vi "XML Script - Tunnel.vi"(2 "out":i32=-1, 3 "default":bool, 4 "location":T1, 6 "name":string, 8 "offset":i32=1, 9 "prefix (name)":string, 10 "in":i32=-1) -> (5 "name (wire source)":string, 7 "XML Script Command - Tunnel":string)   [LabVIEW 2017]
uses:
  <vilib>/_script/XML Scripting/Structure Location.ctl
  <vilib>/_script/XML Scripting/XML Script Tag.ctl
  <vilib>/_script/XML Scripting/XML Script Attribute.ctl
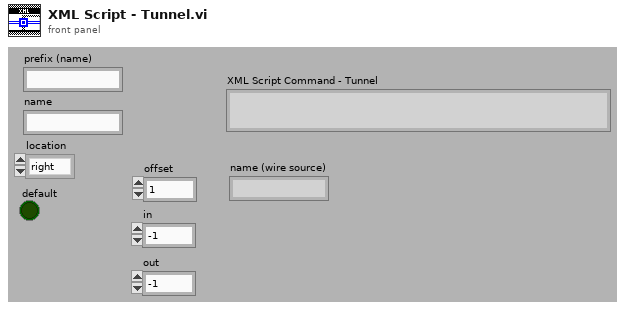
[diagram p1: front panel]
types:
  T1 = typedef "Structure Location.ctl" = enum16{"right", "left", "top", "bottom"}
  T2 = typedef "XML Script Attribute.ctl" = enum16{"name", "style", "path", "position", "in", "out", "width", "height", "index", "value", "default", "location", "offset", "typeindex", "size", "source", "destination", "indicator", "type", "controlname", "label", "conpaneidx", "mode", "description", "hasCondTerm", "linkIdentity", "caseselectortype", "concatInputs", "inName", "instantiationpath", "loopCondition", "IndexMode", "formulaInputs", "formulaOutputs", "msnFuncName", "msnIsDynamic", "msnIsODEUserFunction", "ignoreSearchDialog"}
  T3 = typedef "XML Script Tag.ctl" = enum16{"Script", "Function", "SubVI", "GrowableFunction", "Structure", "MultiframeStructure", "Frame", "Tunnel", "ShiftRegister", "Constant", "Control", "Terminal", "Wire", "StaticVIReference", "ControlTerminal", "CompoundArithmetic", "FlatSequence", "FlatSequenceFrame", "MathScriptCallByRef", "BuildArray", "GenericSubVI", "MathScriptNode"}
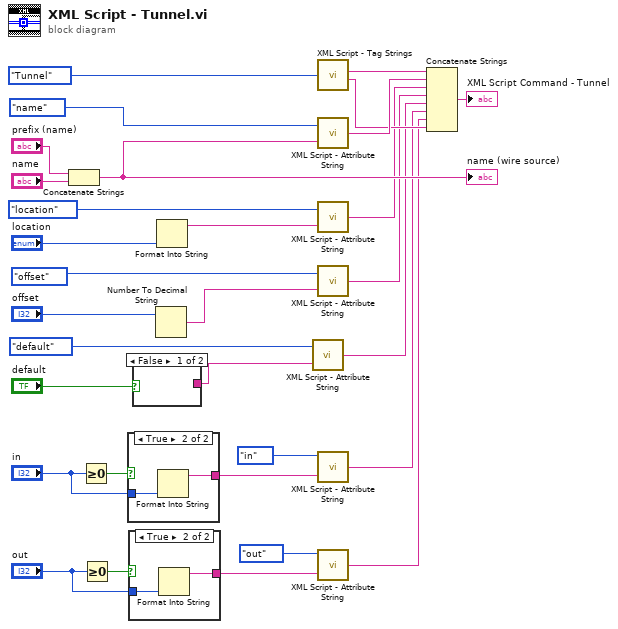
[diagram p0: block diagram]
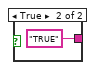
[diagram p2: hidden frame]
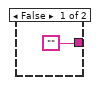
[diagram p3: hidden frame]
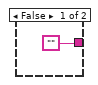
[diagram p4: hidden frame]
diagram:
  n1 = Concatenate Strings("prefix (name)", "name") -> (w21:string)
  "name (wire source)" <- w21
  n2 = Greater Or Equal To 0?(x="in") -> (x >= 0?=w11:bool)
  n3 = Greater Or Equal To 0?(x="out") -> (x >= 0?=w15:bool)
  n4 = case shown="True" w11 {
    tunnel: "in" -> [_ w34]
    tunnel: ["" w33] -> w13
    frame False {
    }
    frame True {
      n5 = Format Into String(w34) -> (resulting string=w33:string)  [unwired: 3 in, 1 out]
    }
  }
  n6 = case shown="True" w15 {
    tunnel: "out" -> [_ w37]
    tunnel: ["" w36] -> w17
    frame False {
    }
    frame True {
      n7 = Format Into String(w37) -> (resulting string=w36:string)  [unwired: 3 in, 1 out]
    }
  }
  n8 = case shown="False" "default" {
    tunnel: [_ "TRUE"] -> w2
    frame False {
    }
    frame True {
    }
  }
  n9 = Number To Decimal String(number="offset") -> (decimal integer string=w18:string)  [unwired: 1 in]
  n10 = Format Into String("location") -> (resulting string=w24:string)  [unwired: 3 in, 1 out]
  n11 = call <vilib>:"XML Script - Attribute String.vi"("Attribute String"=w2, "XML Script Attribute"=XML_Script_Attribute."default") -> ("XML Script - Attribute String"=w1:string)
  n12 = call <vilib>:"XML Script - Tag Strings.vi"("XML Script Tag"=XML_Script_Tag."Tunnel") -> ("XML String - Begin Tag"=w28:string, "XML String - End Tag"=w9:string)  [unwired: 2 in]
  n13 = call <vilib>:"XML Script - Attribute String.vi"("Attribute String"=w21, "XML Script Attribute"=XML_Script_Attribute."name") -> ("XML Script - Attribute String"=w26:string)
  n14 = call <vilib>:"XML Script - Attribute String.vi"("Attribute String"=w24, "XML Script Attribute"=XML_Script_Attribute."location") -> ("XML Script - Attribute String"=w5:string)
  n15 = call <vilib>:"XML Script - Attribute String.vi"("Attribute String"=w18, "XML Script Attribute"=XML_Script_Attribute."offset") -> ("XML Script - Attribute String"=w6:string)
  n16 = call <vilib>:"XML Script - Attribute String.vi"("Attribute String"=w13, "XML Script Attribute"=XML_Script_Attribute."in") -> ("XML Script - Attribute String"=w8:string)
  n17 = call <vilib>:"XML Script - Attribute String.vi"("Attribute String"=w17, "XML Script Attribute"=XML_Script_Attribute."out") -> ("XML Script - Attribute String"=w7:string)
  n18 = Concatenate Strings(w28, w26, w5, w6, w1, w8, w7, w9) -> (→"XML Script Command - Tunnel":string)
